vi "ScreenPop(SubVI).vi"(8 "Error In":errorcluster, 11 "SR #":string) -> (0 "error out":errorcluster)   [LabVIEW 2018, in "DS_Lib.lvlib" / "SRReportParser.lvlib"]
uses:
  SRReportParser.lvlib
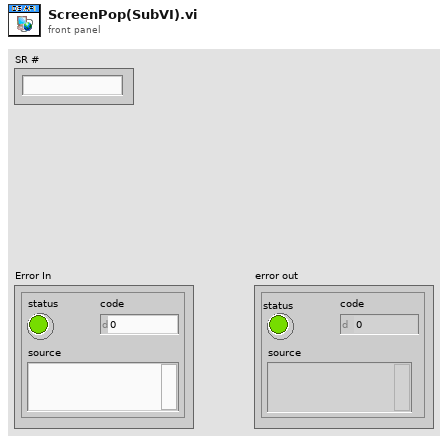
[diagram p1: front panel]
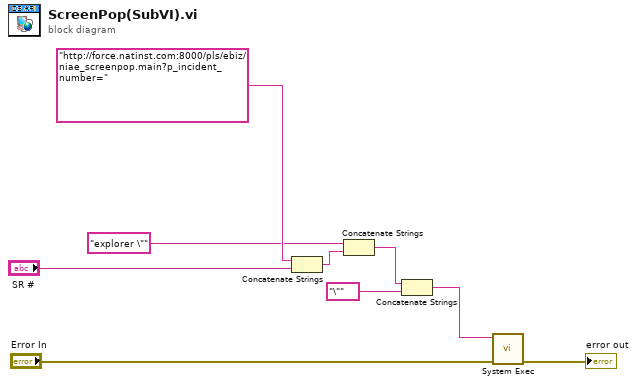
[diagram p0: block diagram]
diagram:
  n1 = Concatenate Strings("http://force.natinst.com:8000/pls/ebiz/niae_screenpop.main?p_incident_number=" ("command line"), "SR #") -> (w8:string)
  n2 = Concatenate Strings("explorer \"" ("string"), w8) -> (w6:string)
  n3 = Concatenate Strings(w6, "\"" ("string")) -> (w4:string)
  n4 = call <vilib>:"System Exec.vi"("error in (no error)"="Error In", "command line"=w4) -> ("error out"=→"error out":errorcluster)  [unwired: 6 in, 3 out]
